vi "Begin.vi"() -> (0 "error out":errorcluster)   [LabVIEW 2012]
doc: "Called before other user functions, this VI is expected to open initial I/O refnums, load in file data, and do all program initialization. Notice that the <B>error out</B> terminal is simply used for data flow. Wiring it to other structures or subVIs ensures that this VI runs first."
uses:
  <vilib>/Rock Robotics/WPI/DriverStation/WPI_DriverStationRobotMode2.ctl
  <vilib>/Rock Robotics/SystemInterfaces/DIO/FPGA_DIOChannel.ctl
  <vilib>/Rock Robotics/WPI/Joystick/WPI_JoystickDeviceEnum.ctl
  <vilib>/Rock Robotics/SystemInterfaces/Typedef/FPGA_TypedefDigitalModule.ctl
  <vilib>/Rock Robotics/SystemInterfaces/DIO/FPGA_DIOPWMChannel.ctl
  Robot Global Data.vi
  <vilib>/Rock Robotics/WPI/Counter/WPI_CounterDigitalInputToDigitalSource.vi
  <vilib>/Rock Robotics/WPI/Counter/WPI_CounterOpen Semi Period Mode.vi
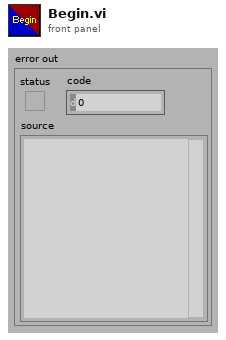
[diagram p1: front panel]
types:
  T1 = typedef "FPGA_DIOPWMChannel.ctl" = enum8{"PWM 1", "PWM 2", "PWM 3", "PWM 4", "PWM 5", "PWM 6", "PWM 7", "PWM 8", "PWM 9", "PWM 10", "Invalid"}
  T2 = typedef "FPGA_DIOChannel.ctl" = enum8{"DIO 1", "DIO 2", "DIO 3", "DIO 4", "DIO 5", "DIO 6", "DIO 7", "DIO 8", "DIO 9", "DIO 10", "DIO 11", "DIO 12", "DIO 13", "DIO 14", "Invalid"}
  T3 = typedef "FPGA_TypedefDigitalModule.ctl" = enum16{"Digital Module 1", "Digital Module 2"}
  T4 = typedef "WPI_JoystickDeviceEnum.ctl" = enum16{"USB 1", "USB 2", "USB 3", "USB 4", "Kinect 1", "Kinect 2"}
  T5 = typedef "WPI_DriverStationRobotMode2.ctl" = enum16{"Autonomous Disabled", "Autonomous Enabled", "Teleop Disabled", "Teleop Enabled", "Timeout", "Finish", "Test Disabled", "Test Enabled"}
  T6 = typedef "WPI_UltrasonicDeviceRef.ctl" = cluster{"DevStatus":errorcluster, "Ping Digital Module":T3, "Echo Digital Module":T3, "Ping Channel":T2, "Echo Channel":T2, "CntIndex":T7}
  T7 = typedef "FPGA_CounterCtrSystemIndex.ctl" = enum8{"Ctr 0", "Ctr 1", "Ctr 2", "Ctr 3", "Ctr 4", "Ctr 5", "Ctr 6", "Ctr 7", "Invalid"}
  T8 = typedef "WPI_DigitalOutputDevRef.ctl" = cluster{"Digital Module":T3, "DIO Channel":T2, "DevStatus":errorcluster}
  T9 = typedef "WPI_DigitalInputDevRef.ctl" = cluster{"DevStatus":errorcluster, "DIO Channel":T2, "Digital Module":T3}
  T10 = typedef "FPGA_CounterEncoderSourceConvertionLVSourceType.ctl" = cluster{"DevStatus":errorcluster, "AnalogTriggerMode?":bool, "DigitalMode":cluster{"Digital Module":T3, "DIO Channel":T11}, "AnalogTriggerMode":cluster{"AnalogTriggerIndex":T12, "OutputType":T13}}
  T11 = typedef "FPGA_DIODigitalSourceChannel.ctl" = enum8{"DIO 1", "DIO 2", "DIO 3", "DIO 4", "DIO 5", "DIO 6", "DIO 7", "DIO 8", "DIO 9", "DIO 10", "DIO 11", "DIO 12", "DIO 13", "DIO 14", "Disabled"}
  T12 = typedef "FPGA_AnalogTriggerIndex.ctl" = enum8{"Trig 0", "Trig 1", "Trig 2", "Trig 3", "Trig 4", "Trig 5", "Trig 6", "Trig 7", "Invalid"}
  T13 = typedef "FPGA_AnalogTriggerOutType.ctl" = enum16{"InWindow", "TriggerState", "Rising", "Falling"}
  T14 = typedef "WPI_CounterDevRef.ctl" = cluster{"DevStatus":errorcluster, "CntIndex":T7}
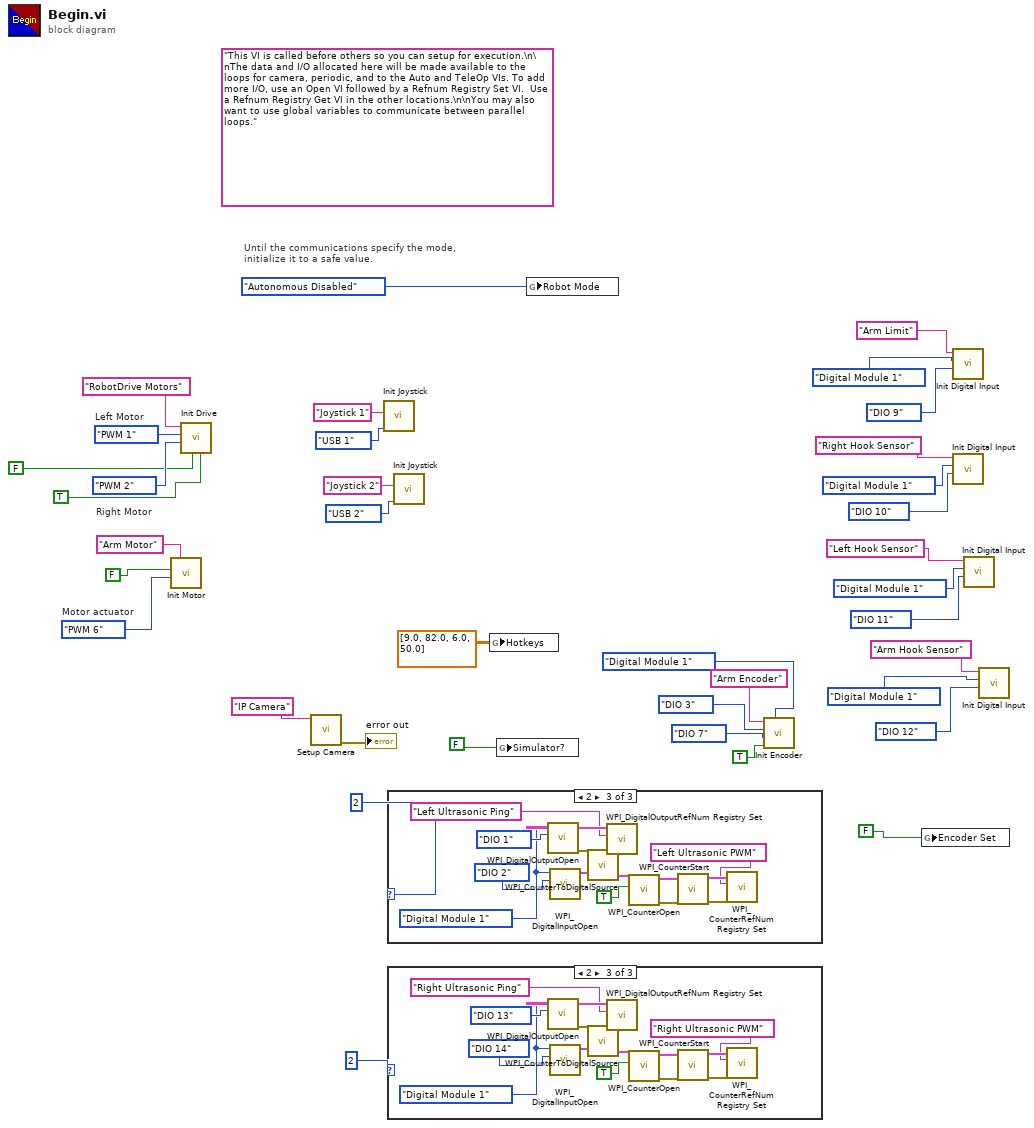
[diagram p0: block diagram]
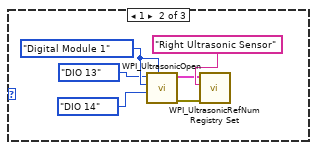
[diagram p3: hidden frame]
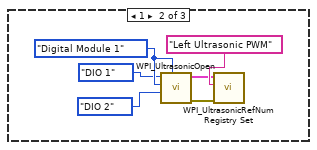
[diagram p5: hidden frame]
diagram:
  w6 = FPGA_DIOPWMChannel."PWM 2"  # Right Motor
  w7 = FPGA_DIOPWMChannel."PWM 1"  # Left Motor
  w11 = FPGA_DIOPWMChannel."PWM 6"  # Motor actuator
  (unwired) "This VI is called before others so you can setup for execution.\n\nThe data and I/O allocated here will be made available to the loops for camera, periodic, and to the Auto and TeleOp VIs. To add more I/O, use an Open VI followed by a Refnum Registry Set VI.  Use a Refnum Registry Get VI in the other locations.\n\nYou may also want to use global variables to communicate between parallel loops."
  # "Until the communications specify the mode,\ninitialize it to a safe value."
  n1 = call "Init Motor.vi"("Motor actuator"=w11, "Motor Actuator Inverted"=FALSE ("Invert Motor"), "refnum name"="Arm Motor") -> ()  [unwired: 9 in]
  n2 = call "Init Drive.vi"("RightMotorInverted"=TRUE, "LeftMotorInverted"=FALSE, "Right Motor"=w6, "Left Motor"=w7, "Drive RefNum"="RobotDrive Motors") -> ()  [unwired: 7 in]
  n3 = call "Setup Camera.vi"("Camera RefNum"="IP Camera") -> ("error out"=→"error out":errorcluster)  [unwired: 10 in]
  n4 = call "Init Joystick.vi"("JoystickDevice"=WPI_JoystickDeviceEnum."USB 1", "Joystick RefNum"="Joystick 1") -> ()  [unwired: 10 in]
  n5 = case shown="2" 2 {
    frame 0, Default {
    }
    frame 1 {
      w43 = FPGA_TypedefDigitalModule."Digital Module 1" ("Digital Module (Module 1)")
      n6 = call <vilib>:"WPI_UltrasonicOpen.vi"("Ping Digital Module (Module 1)"=w43, "Echo DIO Channel"=FPGA_DIOChannel."DIO 2" ("DIO Channel"), "Echo Digital Module (Module 1)"=w43, "Ping DIO Channel"=FPGA_DIOChannel."DIO 1" ("DIO Channel")) -> ("error out"=w40:errorcluster, "UltrasonicDevRef"=w41:T6)  [unwired: 6 in]
      n7 = call <vilib>:"WPI_UltrasonicRefNum Registry Set.vi"("error in (no error)"=w40, "refnum name"="Left Ultrasonic PWM", "UltrasonicDevRef"=w41) -> ()  [unwired: 7 in, 2 out]
    }
    frame 2 {
      w53 = FPGA_TypedefDigitalModule."Digital Module 1" ("Digital Module (Module 1)")
      n8 = call <vilib>:"WPI_DigitalOutputOpen.vi"("DIO Channel"=FPGA_DIOChannel."DIO 1", "Digital Module (Module 1)"=w53) -> ("error out"=w57:errorcluster, "DigitalOutputDevRef"=w56:T8)  [unwired: 8 in]
      n9 = call <vilib>:"WPI_DigitalInputOpen.vi"("DIO Channel"=FPGA_DIOChannel."DIO 2", "Digital Module (Module 1)"=w53) -> ("DigitalInputDevRef"=w51:T9)  [unwired: 8 in, 1 out]
      n10 = call-poly <vilib>:"WPI_CounterToDigitalSource.vi"("DigitalInputDevRef"=w51) -> ("Digital Source"=w50:T10)  [unwired: 6 in]
      n11 = call <vilib>:"WPI_DigitalOutputRefNum Registry Set.vi"("error in (no error)"=w57, "refnum name"="Left Ultrasonic Ping", "DigitalOutputDevRef"=w56) -> ()  [unwired: 7 in, 2 out]
      n12 = call-poly <vilib>:"WPI_CounterOpen.vi"("High Pulse (T)"=TRUE, "Source"=w50) -> ("error out"=w48:errorcluster, "CounterDevRef"=w47:T14)  [unwired: 8 in]
      n13 = call <vilib>:"WPI_CounterStart.vi"("error in (no error)"=w48, "CounterDevRef in"=w47) -> ("error out"=w46:errorcluster, "CounterDevRef out"=w45:T14)  [unwired: 8 in]
      n14 = call <vilib>:"WPI_CounterRefNum Registry Set.vi"("error in (no error)"=w46, "refnum name"="Left Ultrasonic PWM", "CounterDevRef"=w45) -> ()  [unwired: 7 in, 2 out]
    }
  }
  n15 = case shown="2" 2 {
    frame 0, Default {
    }
    frame 1 {
      w63 = FPGA_TypedefDigitalModule."Digital Module 1" ("Digital Module (Module 1)")
      n16 = call <vilib>:"WPI_UltrasonicOpen.vi"("Ping Digital Module (Module 1)"=w63, "Echo DIO Channel"=FPGA_DIOChannel."DIO 14" ("DIO Channel"), "Echo Digital Module (Module 1)"=w63, "Ping DIO Channel"=FPGA_DIOChannel."DIO 13" ("DIO Channel")) -> ("error out"=w60:errorcluster, "UltrasonicDevRef"=w61:T6)  [unwired: 6 in]
      n17 = call <vilib>:"WPI_UltrasonicRefNum Registry Set.vi"("error in (no error)"=w60, "refnum name"="Right Ultrasonic Sensor", "UltrasonicDevRef"=w61) -> ()  [unwired: 7 in, 2 out]
    }
    frame 2 {
      w73 = FPGA_TypedefDigitalModule."Digital Module 1" ("Digital Module (Module 1)")
      n18 = call <vilib>:"WPI_DigitalOutputOpen.vi"("DIO Channel"=FPGA_DIOChannel."DIO 13", "Digital Module (Module 1)"=w73) -> ("error out"=w77:errorcluster, "DigitalOutputDevRef"=w76:T8)  [unwired: 8 in]
      n19 = call <vilib>:"WPI_DigitalInputOpen.vi"("DIO Channel"=FPGA_DIOChannel."DIO 14", "Digital Module (Module 1)"=w73) -> ("DigitalInputDevRef"=w71:T9)  [unwired: 8 in, 1 out]
      n20 = call-poly <vilib>:"WPI_CounterToDigitalSource.vi"("DigitalInputDevRef"=w71) -> ("Digital Source"=w70:T10)  [unwired: 6 in]
      n21 = call <vilib>:"WPI_DigitalOutputRefNum Registry Set.vi"("error in (no error)"=w77, "refnum name"="Right Ultrasonic Ping", "DigitalOutputDevRef"=w76) -> ()  [unwired: 7 in, 2 out]
      n22 = call-poly <vilib>:"WPI_CounterOpen.vi"("High Pulse (T)"=TRUE, "Source"=w70) -> ("error out"=w68:errorcluster, "CounterDevRef"=w67:T14)  [unwired: 8 in]
      n23 = call <vilib>:"WPI_CounterStart.vi"("error in (no error)"=w68, "CounterDevRef in"=w67) -> ("error out"=w66:errorcluster, "CounterDevRef out"=w65:T14)  [unwired: 8 in]
      n24 = call <vilib>:"WPI_CounterRefNum Registry Set.vi"("error in (no error)"=w66, "refnum name"="Right Ultrasonic PWM", "CounterDevRef"=w65) -> ()  [unwired: 7 in, 2 out]
    }
  }
  n25 = call "Init Joystick.vi"("JoystickDevice"=WPI_JoystickDeviceEnum."USB 2", "Joystick RefNum"="Joystick 2") -> ()  [unwired: 10 in]
  n26 = global write "Robot Global Data.vi" "Hotkeys"(dbl[][] [[9.0, 82.0], [6.0, 50.0]] ("Hotkeys")) -> ()
  n27 = global write "Robot Global Data.vi" "Simulator?"(FALSE) -> ()
  n28 = global write "Robot Global Data.vi" "Robot Mode"(WPI_DriverStationRobotMode2."Autonomous Disabled" ("Robot Mode")) -> ()
  n29 = call "Init Encoder.vi"("Digital Module (Module 1)"=FPGA_TypedefDigitalModule."Digital Module 1", "Invert Direction (False)"=TRUE, "DIO Channel 2"=FPGA_DIOChannel."DIO 7" ("DIO Channel 1"), "DIO Channel 1"=FPGA_DIOChannel."DIO 3", "refnum name"="Arm Encoder") -> ()  [unwired: 7 in]
  n30 = global write "Robot Global Data.vi" "Encoder Set"(FALSE) -> ()
  n31 = call "Init Digital Input.vi"("DIO Channel"=FPGA_DIOChannel."DIO 9", "Digital Module"=FPGA_TypedefDigitalModule."Digital Module 1", "Refnum"="Arm Limit") -> ()  [unwired: 8 in, 1 out]
  n32 = call "Init Digital Input.vi"("DIO Channel"=FPGA_DIOChannel."DIO 10", "Digital Module"=FPGA_TypedefDigitalModule."Digital Module 1", "Refnum"="Right Hook Sensor") -> ()  [unwired: 8 in, 1 out]
  n33 = call "Init Digital Input.vi"("DIO Channel"=FPGA_DIOChannel."DIO 11", "Digital Module"=FPGA_TypedefDigitalModule."Digital Module 1", "Refnum"="Left Hook Sensor") -> ()  [unwired: 8 in, 1 out]
  n34 = call "Init Digital Input.vi"("DIO Channel"=FPGA_DIOChannel."DIO 12", "Digital Module"=FPGA_TypedefDigitalModule."Digital Module 1", "Refnum"="Arm Hook Sensor") -> ()  [unwired: 8 in, 1 out]
